vi "Initialize Pump.vi"(4 "Read EU (F)":bool, 6 "Read Backlash (F)":bool, 7 "Pump ID (0:A)":T1, 8 "error in (no error)":errorcluster, 11 "VISA resource in":refnum<visa-resource-name>) -> (0 "error out":errorcluster, 3 "VISA resource out":refnum<visa-resource-name>)   [LabVIEW 2020, in "Global FIA milliGAT.lvlib"]
doc: "Establishes communication with the instrument and optionally performs an instrument identification query and/or an instrument reset. It also places the instrument in a default state needed for other instrument driver operations. Therefore, call this VI before calling other instrument driver VIs for this instrument. Generally, you need to call the <b>Initialize</b> VI only once at the beginning of an application."
uses:
  <instrlib>/RxnRover/Global FIA milliGAT 3.14/Global FIA milliGAT.lvlib
  <instrlib>/RxnRover/Global FIA milliGAT 3.14/Public/Utility/Pump Address.ctl
  <instrlib>/RxnRover/Global FIA milliGAT 3.14/Private/Pump Parameter.ctl
panel:
  # "(c) 2020 Global FIA.  ALL RIGHTS RESERVED."
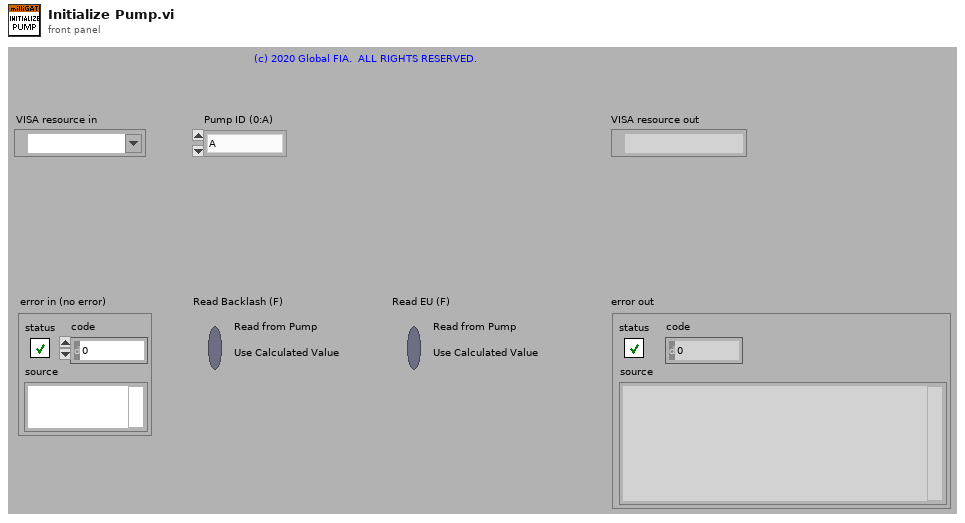
[diagram p1: front panel]
types:
  T1 = typedef "Global FIA milliGAT.lvlib/Pump Address.ctl" = enum16{"A", "B", "C", "D", "E", "F", "G", "H", "I", "J", "K", "L", "M", "N", "O", "P", "Q", "R", "S", "T", "U", "V", "W", "X", "Y", "Z", "a", "b", "c", "d", "e", "f", "g", "h", "i", "j", "k", "l", "m", "n", "o", "p", "q", "r", "s", "t", "u", "v", "w", "x", "y", "z", "0", "1", "2", "3", "4", "5", "6", "7", "8", "9"}
  T2 = typedef "Global FIA milliGAT.lvlib/Pump Parameter.ctl" = enum16{"Enabled", "EU", "EU Calibration Factor", "Fixed Asp or Disp", "Starting Position", "Starting Flow", "Peak Flow", "Flow Acceleration", "Flow Deceleration", "Session Volume", "Max Pressure", "Backlash (usteps)", "BL Calibration Factor", "BL Correction Enabled", "Min Flow", "Max Flow", "Min Acceleration", "Max Acceleration", "Service Volume", "Life Volume"}
  T3 = typedef "Global FIA milliGAT.lvlib/Hardware Configuration.ctl" = cluster{"Head type":enum16{"Low Flow", "High Flow"}, "Pressure range":enum16{"Low pressure", "High pressure"}, "Stator material":enum16{"PTFE", "Valcon E3", "PEEK/PTFE", "Valcon H2"}, "Rotor material":enum16{"Ceramic", "Valcon P", "CTFE"}, "Rotor O-ring material":enum16{"none", "Viton", "Kalrez"}, "Piston O-ring material":enum16{"Viton", "Kalrez"}, "Pump body material":enum16{"Stainless steel", "Aluminum"}, "Controller":enum16{"MForce", "MDrive"}, "Gear ratio":enum16{"4.75", "9.87", "15", "22.56"}, "Motor resolution":enum16{"1.8", "0.9"}, "Equipped with encoder":enum16{"No", "Yes"}}
  T4 = cluster{"EU":dbl, "Backlash (usteps)":dbl, "Max Pressure":dbl, "Min Flow":dbl, "Max Flow":dbl, "Min Acceleration":dbl, "Max Acceleration":dbl, "Service Volume":dbl}
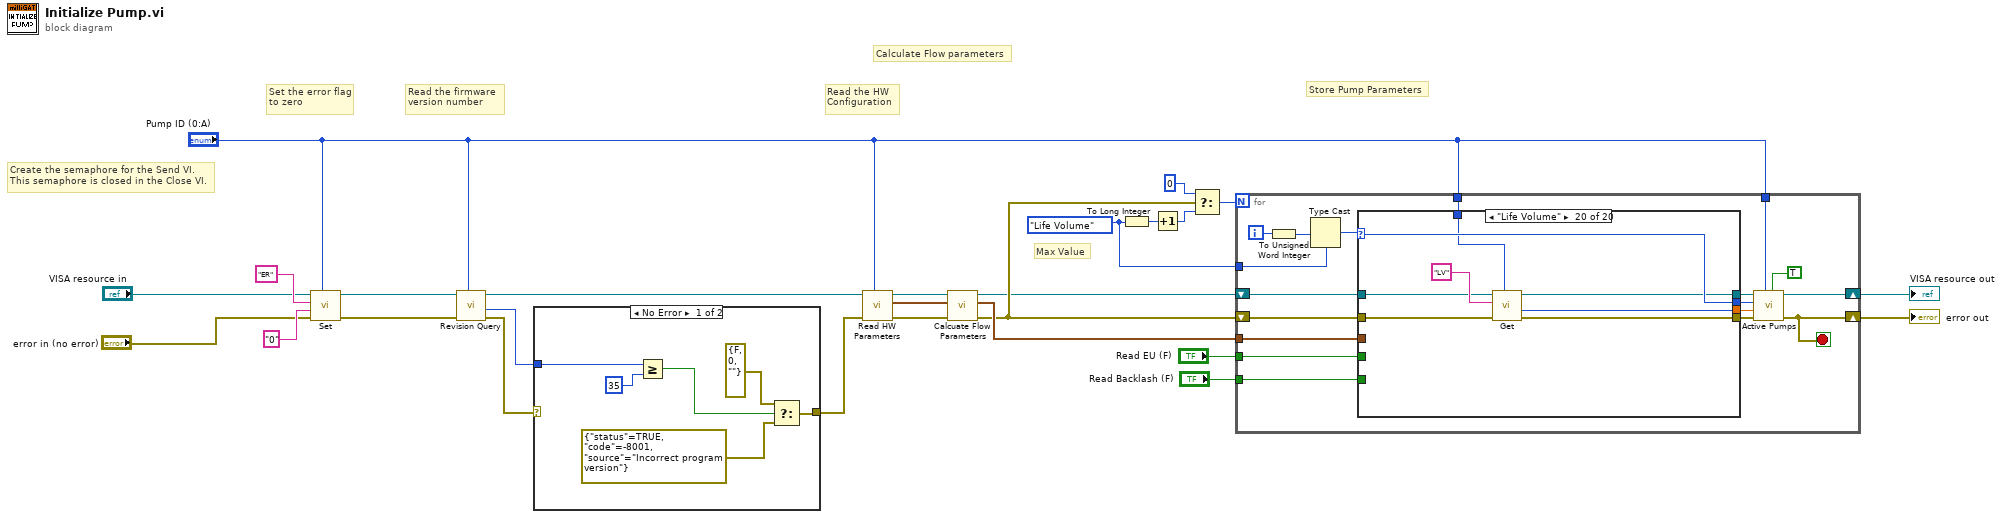
[diagram p0: block diagram]
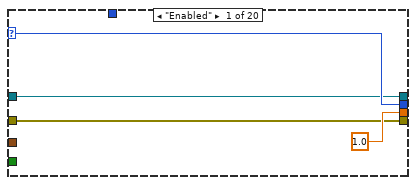
[diagram p2: hidden frame]
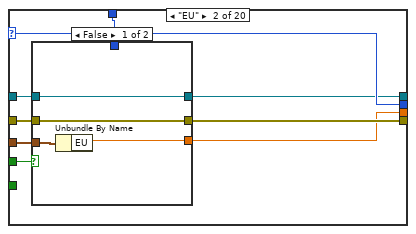
[diagram p3: hidden frame]
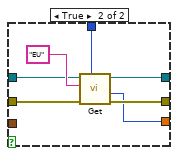
[diagram p4: hidden frame]
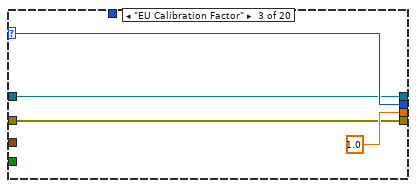
[diagram p5: hidden frame]
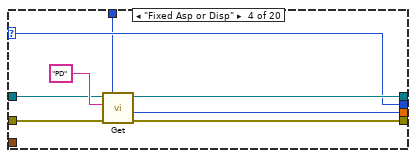
[diagram p6: hidden frame]
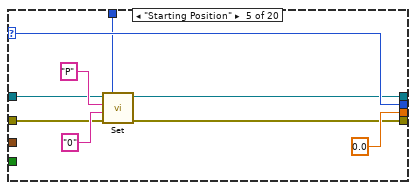
[diagram p7: hidden frame]
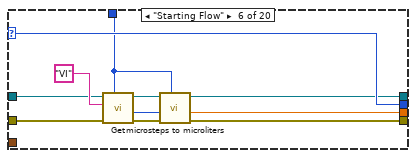
[diagram p8: hidden frame]
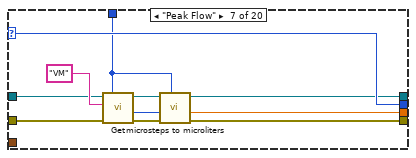
[diagram p9: hidden frame]
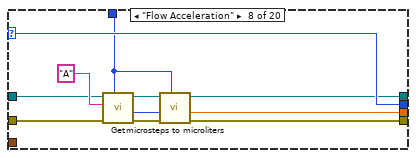
[diagram p10: hidden frame]
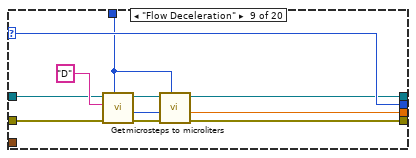
[diagram p11: hidden frame]
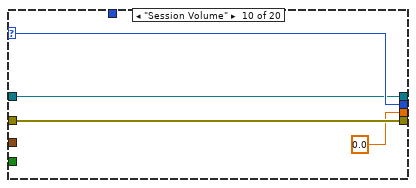
[diagram p12: hidden frame]
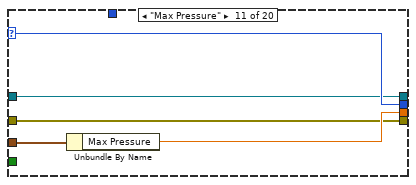
[diagram p13: hidden frame]
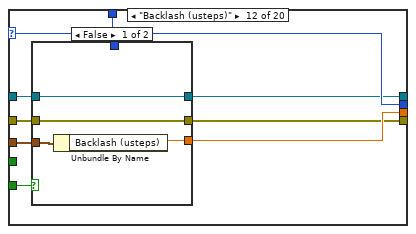
[diagram p14: hidden frame]
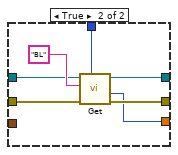
[diagram p15: hidden frame]
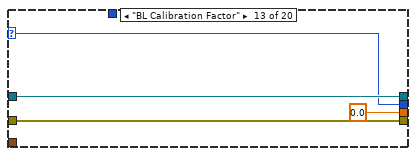
[diagram p16: hidden frame]
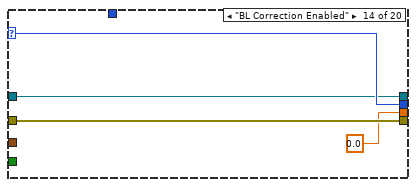
[diagram p17: hidden frame]
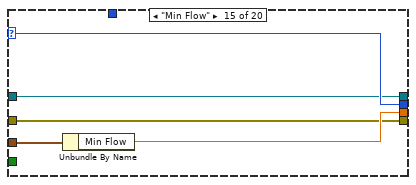
[diagram p18: hidden frame]
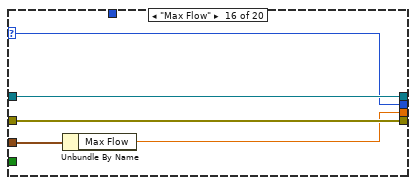
[diagram p19: hidden frame]
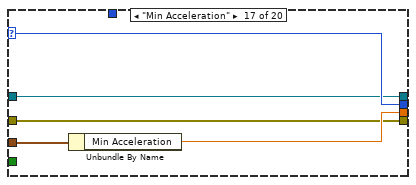
[diagram p20: hidden frame]
diagram:
  w5 = Pump_Parameter."Life Volume" ("Parameter")
  # "Create the semaphore for the Send VI.\nThis semaphore is closed in the Close VI."
  # "Max Value"
  # "Store Pump Parameters"
  # "Calculate Flow parameters"
  # "Read the HW\nConfiguration"
  # "Set the error flag\nto zero"
  # "Read the firmware \nversion number"
  n1 = call <instrlib>:"Set.vi"("Pump ID (0:A)"="Pump ID (0:A)", "error in (no error)"="error in (no error)", "Expression"="0", "Parameter"="ER" ("Parameter Name"), "VISA resource in"="VISA resource in") -> ("error out"=w22:errorcluster, "VISA resource out"=w23:refnum<visa-resource-name>)  [unwired: 5 in]
  n2 = call <instrlib>:"Revision Query.vi"("Pump ID (0:A)"="Pump ID (0:A)", "error in (no error)"=w22, "VISA resource in"=w23) -> ("error out"=w21:errorcluster, "Firmware Revision"=w24:i32, "VISA resource out"=w20:refnum<visa-resource-name>)  [unwired: 5 in, 1 out]
  n3 = case shown="No Error" w21 {
    selector: w21 -> [_ w33]
    tunnel: w24 -> [w28 _]
    tunnel: [w27 w33] -> w19
    frame No Error {
      n4 = Greater Or Equal?(x=w28, y=35) -> (x >= y?=w31:bool)
      n5 = Select(t=errorcluster {"status"=FALSE, "code"=0, "source"=""} ("error out"), s=w31, f=errorcluster {"status"=TRUE, "code"=-8001, "source"="Incorrect program version"}) -> (s? t:f=w27:errorcluster)
    }
    frame Error {
    }
  }
  n6 = call <instrlib>:"Read HW Parameters.vi"("Pump ID (0:A)"="Pump ID (0:A)", "error in (no error)"=w19, "VISA Refnum in"=w20) -> ("error out"=w18:errorcluster, "Hardware Configuration"=w16:T3, "VISA Refnum out"=w17:refnum<visa-resource-name>)  [unwired: 6 in]
  n7 = call <instrlib>:"Calcuate Flow Parameters.vi"("error in (no error)"=w18, "Hardware Configuration"=w16, "VISA resource in"=w17) -> ("error out"=w10:errorcluster, "Flow Configuration"=w15:T4, "VISA resource out"=w9:refnum<visa-resource-name>)  [unwired: 6 in]
  n8 = To Long Integer(number=w5) -> (32bit integer=w4:i32)
  n9 = Increment(x=w4) -> (x+1=w3:i32)
  n10 = Select(t=0, s=w10, f=w3) -> (s? t:f=w14:i32)
  n11 = for {
    N: w14 -> [_]
    tunnel: "Pump ID (0:A)" -> [w43]
    shift-right: [w41] -> w11
    shift-left: w10 -> [w48]
    tunnel: w15 -> [w51]
    shift-right: [w44] -> w12
    shift-left: w9 -> [w49]
    tunnel: "Pump ID (0:A)" -> [w38]
    tunnel: "Read EU (F)" -> [w37]
    tunnel: "Read Backlash (F)" -> [w36]
    tunnel: w5 -> [w34]
    i -> [w40]
    stop <- w41 stop-if-true
    n12 = To Unsigned Word Integer(number=w40) -> (unsigned 16bit integer=w39:u16)
    n13 = Type Cast(type=w34, x=w39) -> (*(type *) &x=w50:T2)
    n14 = case shown="\"Life Volume\"" w50 {
      selector: w50 -> [w55 w64 w79 w83 w94 w102 w113 w124 w135 w140 w146 w156 w169 w175 w179 w182 w189 w193 w198 w207]
      tunnel: w51 -> [_ w63 _ _ _ _ _ _ _ _ w147 w153 _ _ w180 w185 w190 w195 w200 _]
      tunnel: w49 -> [w53 w60 w77 w86 w89 w104 w115 w126 w137 w139 w144 w155 w171 w174 w177 w184 w187 w194 w199 w205]
      tunnel: [w53 w61 w77 w84 w89 w99 w110 w121 w132 w139 w144 w150 w171 w174 w177 w184 w187 w194 w199 w203] -> w45
      tunnel: [w52 w59 w76 w81 w90 w98 w109 w120 w131 w142 w143 w151 w170 w173 w176 w183 w186 w191 w196 w202] -> w46
      tunnel: w48 -> [w52 w58 w76 w85 w90 w103 w114 w125 w136 w142 w143 w154 w170 w173 w176 w183 w186 w191 w196 w204]
      tunnel: [w55 w64 w79 w83 w94 w102 w113 w124 w135 w140 w146 w156 w169 w175 w179 w182 w189 w193 w198 w207] -> w35
      tunnel: [1.0 w57 1.0 w82 0.0 ("Min Acceleration") w96 w107 w118 w129 0.0 ("Min Acceleration") w145 w152 0.0 ("Service Volume") 0.0 ("Service Volume") w178 w181 w188 w192 w197 w201] -> w42
      tunnel: w38 -> [_ w56 _ w80 w88 w95 w106 w117 w128 _ _ w148 _ _ _ _ _ _ _ w206]
      tunnel: w37 -> [_ w62 _ _ _ _ _ _ _ _ _ _ _ _ _ _ _ _ _ _]
      tunnel: w36 -> [_ _ _ _ _ _ _ _ _ _ _ w149 _ _ _ _ _ _ _ _]
      frame "Enabled" {
      }
      frame "EU" {
        n15 = case shown="False" w62 {
          tunnel: w63 -> [w68 _]
          tunnel: [w67 w74] -> w61
          tunnel: w60 -> [w67 w71]
          tunnel: [w66 w73] -> w59
          tunnel: w58 -> [w66 w72]
          tunnel: [w65 w69] -> w57
          tunnel: w56 -> [_ w70]
          frame False {
            n16 = Unbundle By Name(w68) -> ("EU"=w65:dbl)
          }
          frame True {
            n17 = call <instrlib>:"Get.vi"("Pump ID (0:A)"=w70, "error in (no error)"=w72, "Parameter"="EU" ("Parameter or Flag"), "VISA resource in"=w71) -> ("error out"=w73:errorcluster, "Value"=w69:i32, "VISA resource out"=w74:refnum<visa-resource-name>)  [unwired: 5 in]
          }
        }
      }
      frame "EU Calibration Factor" {
      }
      frame "Fixed Asp or Disp" {
        n18 = call <instrlib>:"Get.vi"("Pump ID (0:A)"=w80, "error in (no error)"=w85, "Parameter"="PD" ("Parameter or Flag"), "VISA resource in"=w86) -> ("error out"=w81:errorcluster, "Value"=w82:i32, "VISA resource out"=w84:refnum<visa-resource-name>)  [unwired: 5 in]
      }
      frame "Starting Position" {
        n19 = call <instrlib>:"Set.vi"("Pump ID (0:A)"=w88, "error in (no error)"=w90, "Expression"="0", "Parameter"="P", "VISA resource in"=w89) -> ()  [unwired: 5 in, 2 out]
      }
      frame "Starting Flow" {
        n20 = call <instrlib>:"Get.vi"("Pump ID (0:A)"=w95, "error in (no error)"=w103, "Parameter"="VI" ("Parameter or Flag"), "VISA resource in"=w104) -> ("error out"=w101:errorcluster, "Value"=w97:i32, "VISA resource out"=w100:refnum<visa-resource-name>)  [unwired: 5 in]
        n21 = call <instrlib>:"microsteps to microliters.vi"("Pump ID (0:A)"=w95, "error in (no error)"=w101, "Microsteps (0)"=w97, "VISA resource in"=w100) -> ("error out"=w98:errorcluster, "Microliters"=w96:dbl, "VISA resource out"=w99:refnum<visa-resource-name>)  [unwired: 5 in]
      }
      frame "Peak Flow" {
        n22 = call <instrlib>:"Get.vi"("Pump ID (0:A)"=w106, "error in (no error)"=w114, "Parameter"="VM" ("Parameter or Flag"), "VISA resource in"=w115) -> ("error out"=w112:errorcluster, "Value"=w108:i32, "VISA resource out"=w111:refnum<visa-resource-name>)  [unwired: 5 in]
        n23 = call <instrlib>:"microsteps to microliters.vi"("Pump ID (0:A)"=w106, "error in (no error)"=w112, "Microsteps (0)"=w108, "VISA resource in"=w111) -> ("error out"=w109:errorcluster, "Microliters"=w107:dbl, "VISA resource out"=w110:refnum<visa-resource-name>)  [unwired: 5 in]
      }
      frame "Flow Acceleration" {
        n24 = call <instrlib>:"Get.vi"("Pump ID (0:A)"=w117, "error in (no error)"=w125, "Parameter"="A" ("Parameter or Flag"), "VISA resource in"=w126) -> ("error out"=w123:errorcluster, "Value"=w119:i32, "VISA resource out"=w122:refnum<visa-resource-name>)  [unwired: 5 in]
        n25 = call <instrlib>:"microsteps to microliters.vi"("Pump ID (0:A)"=w117, "error in (no error)"=w123, "Microsteps (0)"=w119, "VISA resource in"=w122) -> ("error out"=w120:errorcluster, "Microliters"=w118:dbl, "VISA resource out"=w121:refnum<visa-resource-name>)  [unwired: 5 in]
      }
      frame "Flow Deceleration" {
        n26 = call <instrlib>:"Get.vi"("Pump ID (0:A)"=w128, "error in (no error)"=w136, "Parameter"="D" ("Parameter or Flag"), "VISA resource in"=w137) -> ("error out"=w134:errorcluster, "Value"=w130:i32, "VISA resource out"=w133:refnum<visa-resource-name>)  [unwired: 5 in]
        n27 = call <instrlib>:"microsteps to microliters.vi"("Pump ID (0:A)"=w128, "error in (no error)"=w134, "Microsteps (0)"=w130, "VISA resource in"=w133) -> ("error out"=w131:errorcluster, "Microliters"=w129:dbl, "VISA resource out"=w132:refnum<visa-resource-name>)  [unwired: 5 in]
      }
      frame "Session Volume" {
      }
      frame "Max Pressure" {
        n28 = Unbundle By Name(w147) -> ("Max Pressure"=w145:dbl)
      }
      frame "Backlash (usteps)" {
        n29 = case shown="False" w149 {
          tunnel: w153 -> [w160 _]
          tunnel: [w159 w166] -> w150
          tunnel: w155 -> [w159 w163]
          tunnel: [w158 w165] -> w151
          tunnel: w154 -> [w158 w164]
          tunnel: [w157 w161] -> w152
          tunnel: w148 -> [_ w162]
          frame False {
            n30 = Unbundle By Name(w160) -> ("Backlash (usteps)"=w157:dbl)
          }
          frame True {
            n31 = call <instrlib>:"Get.vi"("Pump ID (0:A)"=w162, "error in (no error)"=w164, "Parameter"="BL" ("Parameter or Flag"), "VISA resource in"=w163) -> ("error out"=w165:errorcluster, "Value"=w161:i32, "VISA resource out"=w166:refnum<visa-resource-name>)  [unwired: 5 in]
          }
        }
      }
      frame "BL Calibration Factor" {
      }
      frame "BL Correction Enabled" {
      }
      frame "Min Flow" {
        n32 = Unbundle By Name(w180) -> ("Min Flow"=w178:dbl)
      }
      frame "Max Flow" {
        n33 = Unbundle By Name(w185) -> ("Max Flow"=w181:dbl)
      }
      frame "Min Acceleration" {
        n34 = Unbundle By Name(w190) -> ("Min Acceleration"=w188:dbl)
      }
      frame "Max Acceleration" {
        n35 = Unbundle By Name(w195) -> ("Max Acceleration"=w192:dbl)
      }
      frame "Service Volume" {
        n36 = Unbundle By Name(w200) -> ("Service Volume"=w197:dbl)
      }
      frame "Life Volume" {
        n37 = call <instrlib>:"Get.vi"("Pump ID (0:A)"=w206, "error in (no error)"=w204, "Parameter"="LV" ("Parameter or Flag Name"), "VISA resource in"=w205) -> ("error out"=w202:errorcluster, "Value"=w201:i32, "VISA resource out"=w203:refnum<visa-resource-name>)  [unwired: 5 in]
      }
    }
    n38 = call <instrlib>:"Active Pumps.vi"("Action (F:Read)"=TRUE, "Pump ID (0:A)"=w43, "error in (no error)"=w46, "Value in"=w42, "Parameter"=w35, "VISA resource in"=w45) -> ("error out"=w41:errorcluster, "VISA resource out"=w44:refnum<visa-resource-name>)  [unwired: 2 in, 2 out]
  }
  "VISA resource out" <- w12
  "error out" <- w11
